vi "Dialog Box Call.vi"() -> ()   [LabVIEW 2016]
panel:
  in  "Display Message":string="Enter message text."
  in  "Font Name":string="Arial"
  in  "Font Color":u32(colorbox)
  in  "Font Size":u32=22
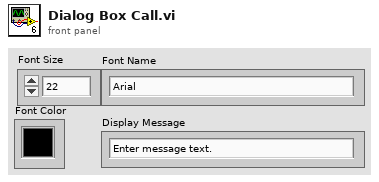
[diagram p1: front panel]
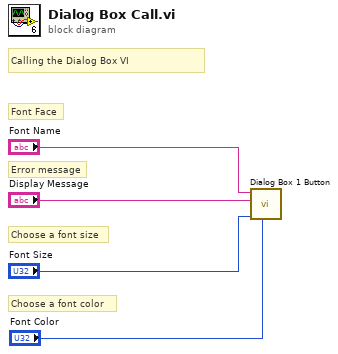
[diagram p0: block diagram]
diagram:
  # "Calling the Dialog Box VI"
  # "Font Face"
  # "Error message"
  # "Choose a font size"
  # "Choose a font color"
  n1 = call "Dialog Box 1 Button.vi"("Font Color"="Font Color", "Font Size"="Font Size", "Input"="Display Message", "Font Name"="Font Name") -> ()  [unwired: 8 in]
